vi "DifferentialFollower SetControl.vi"(0 "DeviceReference":T1, 1 "MasterID":i32, 2 "OpposeMasterDirection":bool, 7 "error in":errorcluster, 18 "Update Frequency (Hz)":dbl=100.0) -> (20 "DeviceReference Out":T1, 27 "error out":errorcluster)   [LabVIEW 2023]
doc: "Follow the differential motor output of another Talon.\nIf Talon is in torque control, the torque is copied - which will increase the total torque applied. If Talon is in percent supply output control, the duty cycle is matched. Motor direction either matches master's configured direction or opposes it based on OpposeMasterDirection."
uses:
  Users/test.DESKTOP-CORY/Documents/PhoenixProLabVIEWGeneration/CopyDown/DeviceReference.ctl
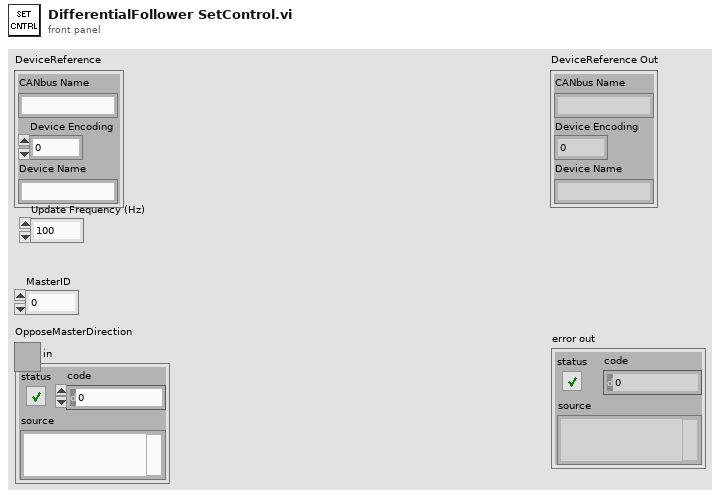
[diagram p1: front panel]
types:
  T1 = typedef "DeviceReference.ctl" = cluster{"CANbus Name":string, "Device Encoding":u32, "Device Name":string}
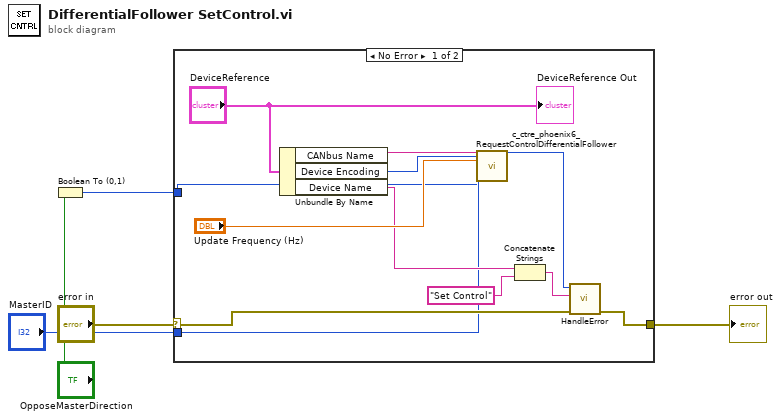
[diagram p0: block diagram]
diagram:
  n1 = Boolean To (0,1)(Boolean="OpposeMasterDirection") -> (0, 1=w1:i16)
  n2 = case shown="No Error" "error in" {
    selector: "error in" -> [w12 w18]
    tunnel: [w11 w18] -> w4
    tunnel: "MasterID" -> [w7 _]
    tunnel: w1 -> [w6 _]
    frame No Error {
      n3 = Unbundle By Name("DeviceReference") -> ("CANbus Name"=w16:string, "Device Encoding"=w15:u32, "Device Name"=w10:string)
      n4 = call <vilib>:"c_ctre_phoenix6_RequestControlDifferentialFollower.vi"("String 2"=w16, "Numeric 2"=w15, "Numeric 3"="Update Frequency (Hz)", "Numeric 5"=w7, 5:w6) -> ("Numeric"=w13:i32)  [unwired: 21 in, 1 out]
      n5 = Concatenate Strings(w10, "Set Control" ("origin")) -> (w8:string)
      n6 = call "HandleError.vi"("error in"=w12, "origin"=w8, "Status"=w13) -> ("error out"=w11:errorcluster)  [unwired: 8 in]
      "DeviceReference Out" <- "DeviceReference"
    }
    frame Error {
    }
  }
  "error out" <- w4
